vi "Save_Images_fr_iSpy.vi"(2 "No Of Attempts":i32=10) -> (0 "Error out":errorcluster)   [LabVIEW 2020]
uses:
  Anemometry/Anemometry Sub Vis/Globals/Meas_global.vi
  Anemometry/Anemometry Sub Vis/Globals/Extra_Commands_Global.vi
  Globals/CamServer global.vi
  Anemometry/Anemometry Sub Vis/Globals/Constants_global.vi
  Anemometry/Anemometry Sub Vis/Globals/Trav_pos_global.vi
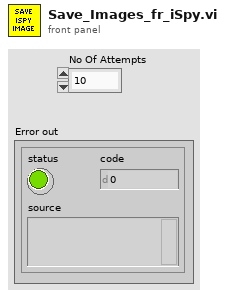
[diagram p1: front panel]
types:
  T1 = typedef "Camera enum.ctl" = string
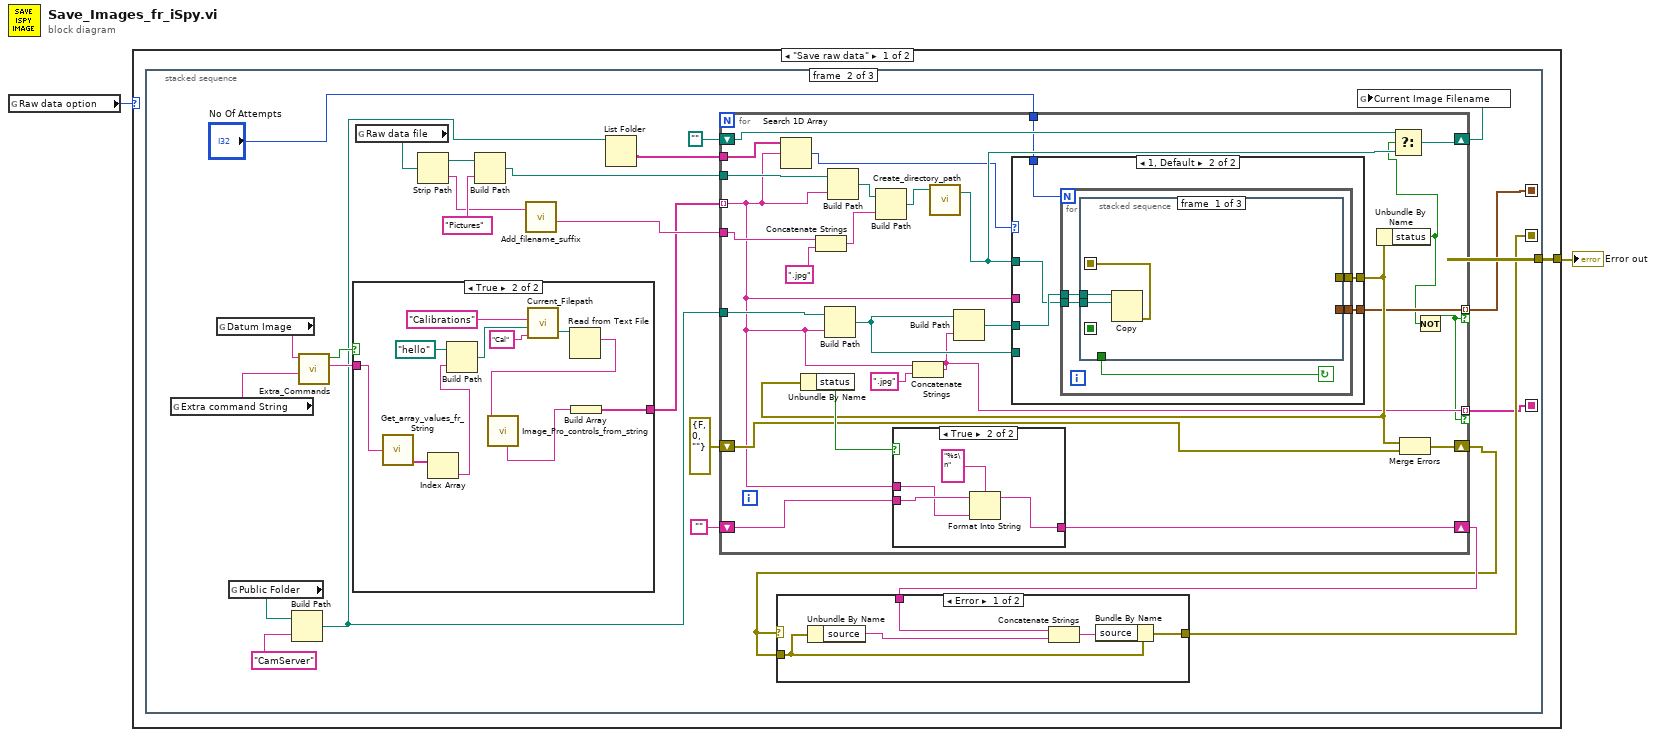
[diagram p0: block diagram]
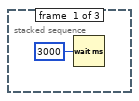
[diagram p2: hidden frame]
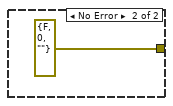
[diagram p3: hidden frame]
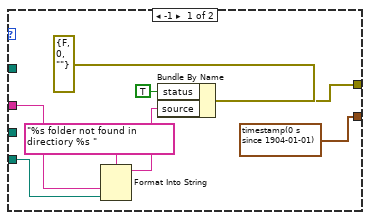
[diagram p4: hidden frame]
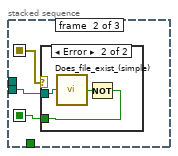
[diagram p5: hidden frame]
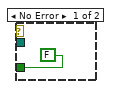
[diagram p6: hidden frame]
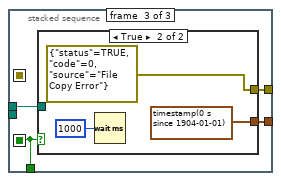
[diagram p7: hidden frame]
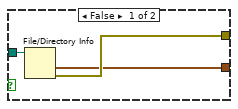
[diagram p8: hidden frame]
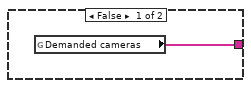
[diagram p10: hidden frame]
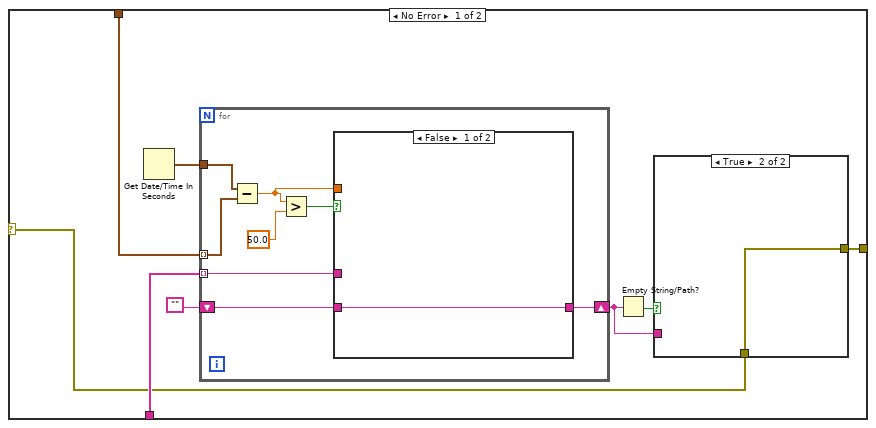
[diagram p12: hidden frame]
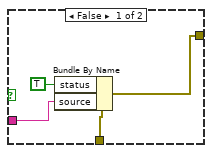
[diagram p13: hidden frame]
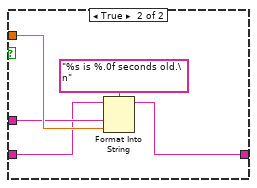
[diagram p14: hidden frame]
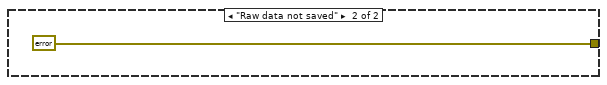
[diagram p15: hidden frame]
diagram:
  n1 = global read "Meas_global.vi" "Raw data option"() -> (w2:enum16{"Save raw data", "Raw data not saved"})
  n2 = case shown="\"Save raw data\"" w2 {
    tunnel: [w3 errorcluster {"status"=FALSE, "code"=0, "source"=""} ("Error out")] -> w1
    frame "Save raw data" {
      n3 = stacked-sequence {
        seq-local: [_ w8 _] -> [_ _ w121]
        seq-local: [_ w7 _] -> [_ _ w120]
        seq-local: [_ w6 _] -> [_ _ w119]
        tunnel: [_ _ w118] -> w3
        frame #0 {
          n4 = Wait (ms)(milliseconds to wait=u32 3000) -> ()  [unwired: 1 out]
        }
        frame #1 {
          n5 = global read "Meas_global.vi" "Extra command String"() -> (w20:string)
          n6 = global read "Extra_Commands_Global.vi" "Datum Image"() -> (w24:string)
          n7 = global read "Constants_global.vi" "Public Folder"() -> (w12:path)
          n8 = Build Path(base path=w12, name or relative path="CamServer") -> (appended path=w9:path)
          n9 = call "Extra_Commands.vi"("String to Search"=w20, "Command"=w24) -> ("String Value"=w21:string, "Command Found"=w23:bool)  [unwired: 2 in, 2 out]
          n10 = case shown="True" w23 {
            tunnel: [w106 w112] -> w22
            tunnel: w21 -> [_ w108]
            frame False {
              n11 = global read "CamServer global.vi" "Demanded cameras"() -> (w106:T1[])
            }
            frame True {
              n12 = call "Get_array_values_fr_String.vi"("String Value"=w108) -> ("String array"=w109:string[])  [unwired: 1 out]
              n13 = Index Array(array=w109) -> (element=w107:string)  [unwired: 1 in]
              n14 = Build Path(base path=path "hello", name or relative path=w107) -> (appended path=w113:path)
              n15 = call "Current_Filepath.vi"("Short_Name"="Cal" ("Data Type"), "Filename in"=w113, "Data Type"="Calibrations") -> ("Filename Out"=w117:path)  [unwired: 1 in, 1 out]
              n16 = Read from Text File(file (use dialog)=w117) -> (text=w111:string)  [unwired: 3 in, 3 out]
              n17 = call "Image_Pro_controls_from_string.vi"("Setup String"=w111) -> ("Camera"=w110:string)  [unwired: 6 in, 4 out]
              n18 = Build Array(w110) -> (w112:string[])
            }
          }
          n19 = global read "Meas_global.vi" "Raw data file"() -> (w27:path)
          n20 = Strip Path(path=w27) -> (stripped path=w29:path, name=w26:string)
          n21 = Build Path(base path=w29, name or relative path="Pictures") -> (appended path=w11:path)
          n22 = call "Add_filename_suffix.vi"("Filename"=w26) -> ("Base name"=w25:string)  [unwired: 1 in, 3 out]
          n23 = List Folder(path=w9) -> (folder names=w10:string[])  [unwired: 3 in, 3 out]
          n24 = for {
            tunnel: w25 -> [w52]
            tunnel: w22 -> [w42] mode=indexing
            shift-right: [w61] -> w18
            shift-left: "" -> [w60]
            shift-right: [w58] -> w16
            shift-left: path "" -> [w59]
            shift-right: [w56] -> w14
            shift-left: errorcluster {"status"=FALSE, "code"=0, "source"=""} ("error IO") -> [w57]
            tunnel: w11 -> [w55]
            tunnel: w9 -> [w49]
            tunnel: w10 -> [w44]
            tunnel: [w40] -> w7 mode=indexing if=w37
            tunnel: [w38] -> w6 mode=indexing if=w37
            tunnel: "No Of Attempts" -> [w36]
            n25 = Search 1D Array(1D array=w44, element=w42) -> (index of element=w43:i32)  [unwired: 1 in]
            n26 = Concatenate Strings(w52, ".jpg" ("string")) -> (w51:string)
            n27 = Build Path(base path=w49, name or relative path=w42) -> (appended path=w41:path)
            n28 = Build Path(base path=w55, name or relative path=w42) -> (appended path=w54:path)
            n29 = Build Path(base path=w54, name or relative path=w51) -> (appended path=w50:path)
            n30 = Concatenate Strings(w42, ".jpg" ("string")) -> (w38:string)
            n31 = call "Create_directory_path.vi"("Path name"=w50) -> ("Path name Out"=w45:path)  [unwired: 2 in, 1 out]
            n32 = Build Path(base path=w41, name or relative path=w38) -> (appended path=w47:path)
            n33 = case shown="1, Default" w43 {
              tunnel: w47 -> [_ w75]
              tunnel: [w69 w74] -> w46
              tunnel: w45 -> [_ w73]
              tunnel: w42 -> [w67 _]
              tunnel: w41 -> [w64 _]
              tunnel: [timestamp(0 s since 1904-01-01) ("last mod") w72] -> w40
              tunnel: w36 -> [_ w71]
              frame -1 {
                n34 = Format Into String(format string="%s folder not found in directiory %s ", w67, w64) -> (resulting string=w66:string)  [unwired: 2 in, 1 out]
                n35 = Bundle By Name(cluster=errorcluster {"status"=FALSE, "code"=0, "source"=""} ("error out"), "status"=TRUE, "source"=w66) -> (w69:errorcluster)
              }
              frame 1, Default {
                n36 = for {
                  N: w71 -> [_]
                  tunnel: w75 -> [w80]
                  tunnel: [w77] -> w74
                  tunnel: w73 -> [w79]
                  tunnel: [w76] -> w72
                  stop <- w78 continue-if-true
                  n37 = stacked-sequence {
                    seq-local: [w81 _ _] -> [_ w86 _]
                    seq-local: [_ w85 _] -> [_ _ w94]
                    tunnel: w80 -> [w83 _ w93]
                    tunnel: w79 -> [w82 w84 _]
                    tunnel: [_ _ w94] -> w78
                    tunnel: [_ _ w92] -> w77
                    tunnel: [_ _ w91] -> w76
                    frame #0 {
                      n38 = Copy(10:w82, 11:w83) -> (0:w81:errorcluster)  [unwired: 3 in, 2 out]
                    }
                    frame #1 {
                      n39 = case shown="Error" w86 {
                        tunnel: [FALSE w88] -> w85
                        tunnel: w84 -> [_ w90]
                        frame No Error {
                        }
                        frame Error {
                          n40 = call "Does_file_exist_(simple).vi"("Pathname"=w90) -> ("exists?"=w89:bool)
                          n41 = Not(x=w89) -> (.not. x?=w88:bool)
                        }
                      }
                    }
                    frame #2 {
                      n42 = case shown="True" w94 {
                        tunnel: w93 -> [w97 _]
                        tunnel: [w96 errorcluster {"status"=TRUE, "code"=0, "source"="File Copy Error"} ("error out")] -> w92
                        tunnel: [w95 timestamp(0 s since 1904-01-01) ("last mod")] -> w91
                        frame False {
                          n43 = File/Directory Info(path=w97) -> (last mod=w95:timestamp, error out=w96:errorcluster)  [unwired: 1 in, 5 out]
                        }
                        frame True {
                          n44 = Wait (ms)(milliseconds to wait=u32 1000) -> ()  [unwired: 1 out]
                        }
                      }
                    }
                  }
                }
              }
            }
            n45 = Unbundle By Name(w46) -> ("status"=w62:bool)
            n46 = case shown="True" w62 {
              tunnel: [w101 w103] -> w61
              tunnel: w60 -> [w101 w105]
              tunnel: w42 -> [_ w104]
              frame False {
              }
              frame True {
                n47 = Format Into String(format string="%s\n", initial string=w105, w104) -> (resulting string=w103:string)  [unwired: 1 in, 1 out]
              }
            }
            n48 = Unbundle By Name(w46) -> ("status"=w39:bool)
            n49 = Select(t=w59, s=w39, f=w45) -> (s? t:f=w58:path)
            n50 = Merge Errors(w46, w57) -> (w56:errorcluster)
            n51 = Not(x=w39) -> (.not. x?=w37:bool)
          }
          n52 = case shown="Error" w14 {
            tunnel: [w33 errorcluster {"status"=FALSE, "code"=0, "source"=""} ("Error out")] -> w8
            tunnel: w18 -> [w32 _]
            tunnel: w14 -> [w34 _]
            frame Error {
              n53 = Unbundle By Name(w34) -> ("source"=w31:string)
              n54 = Concatenate Strings(w32, w31) -> (w30:string)
              n55 = Bundle By Name(cluster=w34, "source"=w30) -> (w33:errorcluster)
            }
            frame No Error {
            }
          }
          n56 = global write "Trav_pos_global.vi" "Current Image Filename"(w16) -> ()
        }
        frame #2 {
          n57 = case shown="Error" w121 {
            selector: w121 -> [w125 w149]
            tunnel: w120 -> [w129 _]
            tunnel: w119 -> [w127 _]
            tunnel: [w123 w149] -> w118
            frame No Error {
              n58 = Get Date/Time In Seconds() -> (seconds since 1Jan1904=w128:timestamp)
              n59 = for {
                tunnel: w129 -> [w141] mode=indexing
                tunnel: w128 -> [w142]
                tunnel: w127 -> [w137] mode=indexing
                shift-right: [w135] -> w122
                shift-left: "" -> [w136]
                n60 = Subtract(x=w142, y=w141) -> (x-y=w139:dbl)
                n61 = Greater?(x=w139, y=50.0) -> (0:w138:bool)
                n62 = case shown="False" w138 {
                  tunnel: w139 -> [_ w148]
                  tunnel: w137 -> [_ w147]
                  tunnel: w136 -> [w143 w145]
                  tunnel: [w143 w144] -> w135
                  frame False {
                  }
                  frame True {
                    n63 = Format Into String(format string="%s is %.0f seconds old.\n", initial string=w145, w147, w148) -> (resulting string=w144:string)  [unwired: 1 in, 1 out]
                  }
                }
              }
              n64 = Empty String/Path?(string/path=w122) -> (empty?=w124:bool)
              n65 = case shown="True" w124 {
                tunnel: w125 -> [w133 w134]
                tunnel: [w132 w134] -> w123
                tunnel: w122 -> [w131 _]
                frame False {
                  n66 = Bundle By Name(cluster=w133, "status"=TRUE, "source"=w131) -> (w132:errorcluster)
                }
                frame True {
                }
              }
            }
            frame Error {
            }
          }
        }
      }
    }
    frame "Raw data not saved" {
    }
  }
  "Error out" <- w1
